vi "filepath global variable.vi"() -> ()   [LabVIEW 2024]
panel:
  in  "awg test waveform":path=path "C:/Users/Mikamilab/Documents/lightsheet/LabVIEW3D/AWGfor3D/waveformforalignment.rd16"
  in  "save_path.txt":path=path "\\\\DESKTOP-8MK9BQ0\\Users/mlab-/Documents/Github-shishido/Closed-loop-optogenetics/xyStage/log/save_path.txt"
  in  "save_time.txt":path=path "\\\\DESKTOP-8MK9BQ0\\Users/mlab-/Documents/Github-shishido/Closed-loop-optogenetics/xyStage/log/start_time.txt"
  in  "img save folder (slave)":path=path "E:/"
  in  "pico temp":path=path "\\\\169.254.104.216\\E:/test.pico"
  in  "img save folder":path=path "E:/"
  in  "xy pixsize label":string="xy pixsize [um]"
  in  "FGconfig for slave":path=path "\\\\169.254.104.216\\Documents/lightsheet/LabVIEW3D/camsetup.csv"
  in  "FGconfig":path=path "\\\\169.254.104.216\\Documents/lightsheet/LabVIEW3D/config"
  in  "masterPC filesave":path=path "\\\\169.254.104.216\\e"
  in  "g1fit":path=path "E:/g1fitcalib"
  in  ".calib":path=path "E:/calibration"
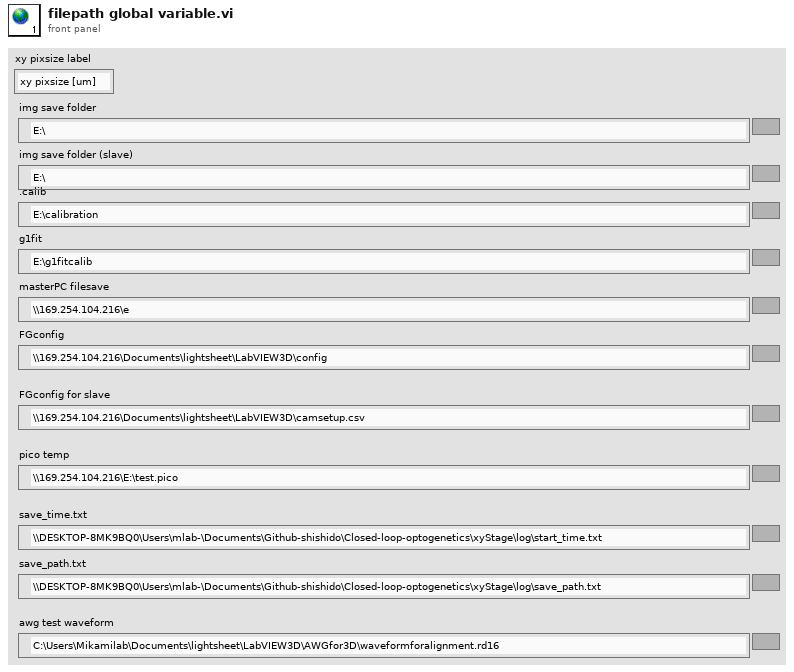
[diagram p1: front panel]
diagram:
